vi "oa_Calculate Continuous Angular Speed.vi"(7 "reset? (True)":bool=TRUE, 8 "error in (no error)":errorcluster, 9 "filter coefficients":dbl[](array[numeric]) format="%.2f", 10 "deltaX":dbl=1.0 format="%.2f", 11 "Y[n]":dbl[](array[numeric]) format="%.2f") -> (0 "error out":errorcluster, 2 "dY/dX[n]":dbl[](array[numeric]) format="%.2f", 3 "pulse out":dbl[](array[numeric]) format="%.2f")   [LabVIEW 2017, in "SoundVib_TachProcess.lvlib"]
uses:
  <vilib>/addons/Sound and Vibration/Order Analysis/Tach Process/SoundVib_TachProcess.lvlib
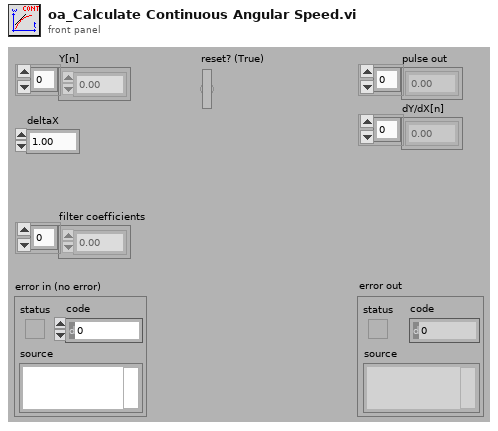
[diagram p1: front panel]
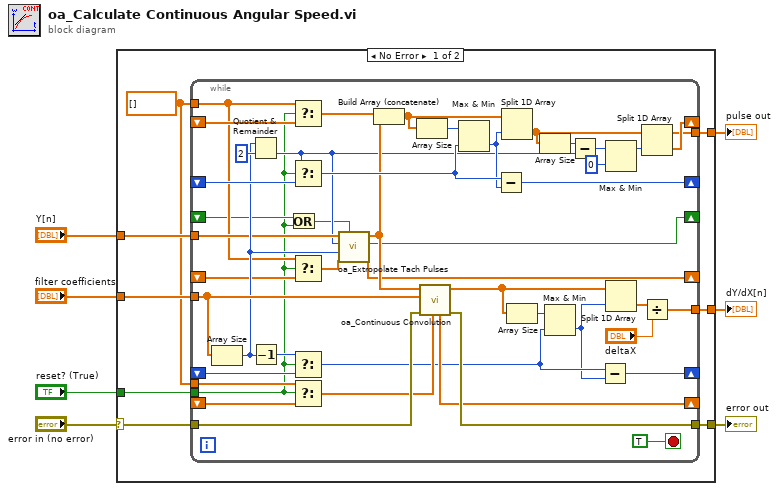
[diagram p0: block diagram]
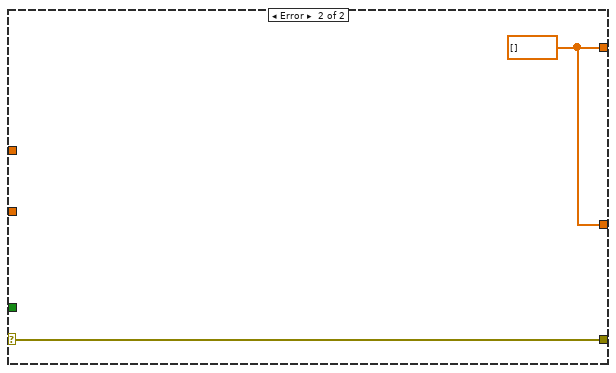
[diagram p2: hidden frame]
diagram:
  n1 = case shown="No Error" "error in (no error)" {
    selector: "error in (no error)" -> [w13 w63]
    tunnel: [w15 w63] -> w7
    tunnel: [w14 w62] -> w6
    tunnel: [w9 w62] -> w5
    tunnel: "Y[n]" -> [w11 _]
    tunnel: "filter coefficients" -> [w12 _]
    tunnel: "reset? (True)" -> [w10 _]
    frame No Error {
      w8 = dbl[] [] ("t")
      n2 = while {
        tunnel: [w61] -> w15
        tunnel: [w60] -> w14
        tunnel: w13 -> [w58]
        tunnel: w12 -> [w53]
        tunnel: w11 -> [w25]
        shift-right: [w54] -> _
        shift-left: _ -> [w56]
        shift-right: [w42] -> _
        shift-left: _ -> [w39]
        shift-right: [w48] -> _
        shift-left: _ -> [w47]
        tunnel: w10 -> [w17]
        tunnel: [w41] -> w9
        tunnel: w8 -> [w20]
        shift-right: [w30] -> _
        shift-left: _ -> [w36]
        shift-right: [w26] -> _
        shift-left: _ -> [w22]
        tunnel: w8 -> [w23]
        shift-right: [w19] -> _
        shift-left: _ -> [w18]
        stop <- TRUE stop-if-true
        n3 = Array Size(array=w53) -> (size(s)=w29:i32)
        n4 = Quotient & Remainder(x=w29, y=2) -> (floor(x/y)=w24:i32)  [unwired: 1 out]
        n5 = Decrement(x=w29) -> (x-1=w37:i32)
        n6 = Or(x=w18, y=w17) -> (x .or. y?=w16:bool)
        n7 = Select(t=w20, s=w17, f=w39) -> (s? t:f=w38:dbl[])
        n8 = Select(t=w24, s=w17, f=w47) -> (s? t:f=w50:i32)
        n9 = Select(t=w20, s=w17, f=w22) -> (s? t:f=w21:dbl[])
        n10 = Select(t=w37, s=w17, f=w36) -> (s? t:f=w32:i32)
        n11 = Select(t=w23, s=w17, f=w56) -> (s? t:f=w55:dbl[])
        n12 = call <vilib>:"oa_Extropolate Tach Pulses.vi"("reset? (True)"=w16, "pulse buffer in"=w21, "modal length"=w29, "extrapolation length"=w24, "pulse in"=w25) -> ("pulse buffer out"=w26:dbl[], "not enough pulses?"=w19:bool, "pulse out"=w28:dbl[])  [unwired: 4 in]
        n13 = Build Array (concatenate)(w38, w28) -> (w40:dbl[])
        n14 = Array Size(array=w40) -> (size(s)=w51:i32)
        n15 = call <vilib>:"oa_Continuous Convolution.vi"("initial state"=w55, "error in (no error)"=w58, "filter coefficients"=w53, "X"=w28) -> ("error out"=w61:errorcluster, "Y"=w35:dbl[], "final state"=w54:dbl[])  [unwired: 5 in]
        n16 = Max & Min(x=w51, y=w50) -> (min(x,y)=w49:i32)  [unwired: 1 out]
        n17 = Subtract(x=w50, y=w49) -> (x-y=w48:i32)
        n18 = Split 1D Array(array=w40, index=w49) -> (second subarray=w46:dbl[])  [unwired: 1 out]
        n19 = Array Size(array=w35) -> (size(s)=w34:i32)
        n20 = Array Size(array=w46) -> (size(s)=w45:i32)
        n21 = Max & Min(x=w34, y=w32) -> (min(x,y)=w31:i32)  [unwired: 1 out]
        n22 = Subtract(x=w45, y=w24) -> (x-y=w44:i32)
        n23 = Subtract(x=w32, y=w31) -> (x-y=w30:i32)
        n24 = Max & Min(x=w44, y=0) -> (max(x,y)=w27:i32)  [unwired: 1 out]
        n25 = Split 1D Array(array=w35, index=w31) -> (second subarray=w33:dbl[])  [unwired: 1 out]
        n26 = Split 1D Array(array=w46, index=w27) -> (first subarray=w41:dbl[], second subarray=w42:dbl[])
        n27 = Divide(x=w33, y="deltaX") -> (x/y=w60:dbl[])
      }
    }
    frame Error {
      w62 = dbl[] []
    }
  }
  "dY/dX[n]" <- w6
  "error out" <- w7
  "pulse out" <- w5
